vi "valve_control_output_tester.vi"(0 "STOP! Refnum":refnum<vi>, 2 "Voltage Arr Refnum":refnum<vi>, 3 "Startup Voltages":dbl[](array[numeric]), 4 "Liquid channel":tag="cDAQ1Mod4/ao3", 5 "Vapor channel":tag="cDAQ1Mod4/ao2") -> ()   [LabVIEW 2017]
uses:
  <vilib>/DAQmx/write.llb/DAQmx Write (Analog 1D Wfm NChan NSamp).vi
  <vilib>/DAQmx/create/channels.llb/DAQmx Create Channel (AO-Voltage-Basic).vi
  <vilib>/DAQmx/configure/timing.llb/DAQmx Timing (Sample Clock).vi
  <vilib>/DAQmx/miscellaneous.llb/DAQmx Fill In Error Info.vi
  <resource>/objmgr/daqmx.rc
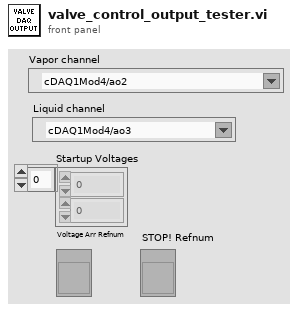
[diagram p1: front panel]
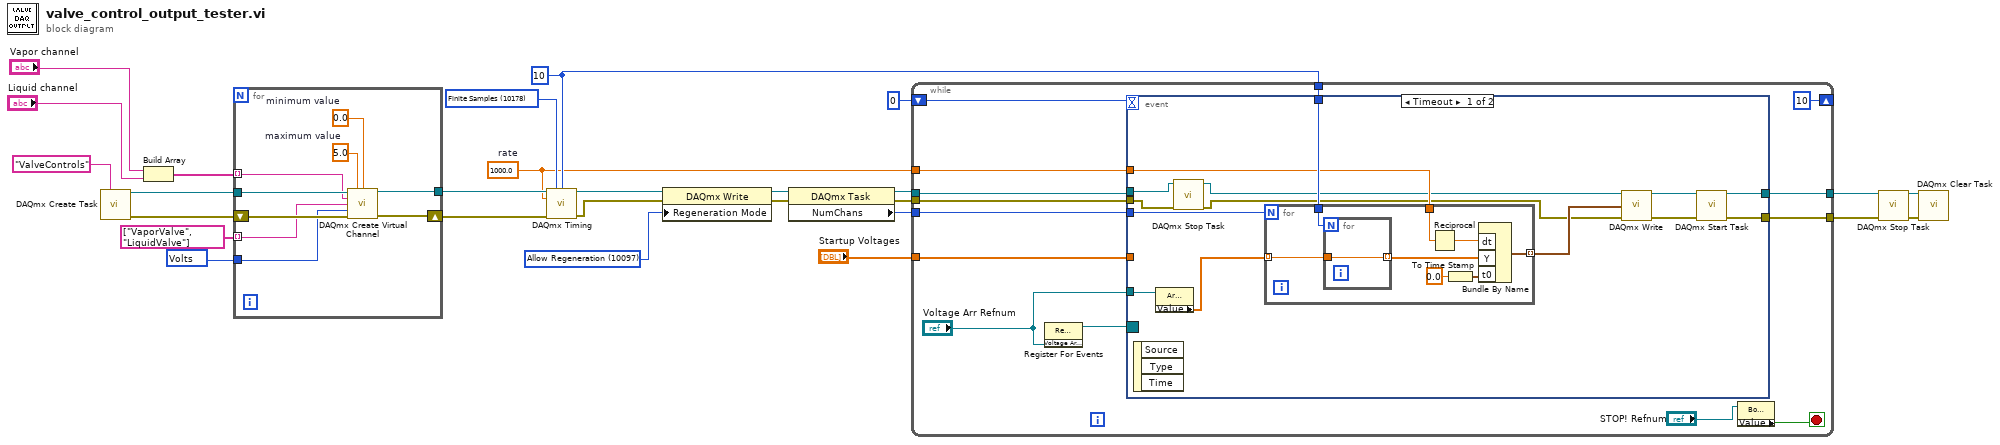
[diagram p0: block diagram]
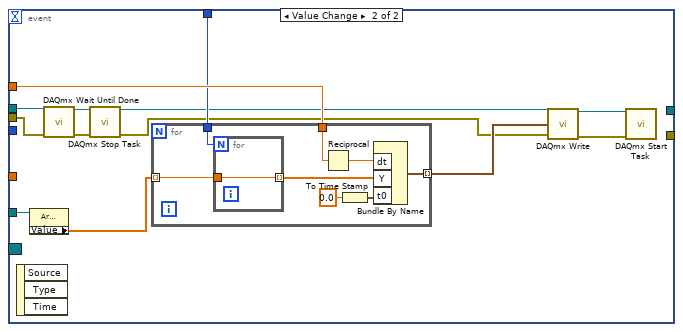
[diagram p2: hidden frame]
diagram:
  w14 = 10097 items=["Allow Regeneration"=10097, "Do Not Allow Regeneration"=10158] ("RegenMode")
  w9 = 10 ("samples per channel")
  w17 = 10178 items=["Finite Samples"=10178, "Continuous Samples"=10123, "Hardware Timed Single Point"=12522] ("sample mode")
  w8 = 1000.0  # rate
  w23 = 10348 items=["Volts"=10348, "From Custom Scale"=10065] ("units")
  n1 = call <vilib>:"DAQmx Create Task.vi"("new task name"="ValveControls") -> ("task out"=w26:refnum<k21>, "error out"=w25:errorcluster)  [unwired: 13 in]
  n2 = Build Array("Vapor channel", "Liquid channel") -> (w20:tag[])
  n3 = for {
    tunnel: w26 -> [w36]
    shift-right: [w28] -> w18
    shift-left: w25 -> [w35]
    tunnel: string[] ["VaporValve", "LiquidValve"] -> [w34] mode=indexing
    tunnel: w23 -> [w33]
    tunnel: w20 -> [w32] mode=indexing
    tunnel: [w29] -> w19
    w30 = 0.0  # minimum value
    w31 = 5.0  # maximum value
    n4 = call-poly <vilib>:"DAQmx Create Virtual Channel.vi"("task in"=w36, "maximum value"=w31, "minimum value"=w30, "physical channels"=w32, "name to assign"=w34, "units"=w33, "error in"=w35) -> ("task out"=w29:refnum<k21>, "error out"=w28:errorcluster)  [unwired: 7 in]
  }
  n5 = call-poly <vilib>:"DAQmx Timing.vi"("task/channels in"=w19, "sample mode"=w17, "samples per channel"=w9, "rate"=w8, "error in"=w18) -> ("task out"=w16:refnum<k21>, "error out"=w15:errorcluster)  [unwired: 9 in]
  n6 = property class="DAQmx Write"(reference=w16, error in=w15, "Regeneration Mode"=w14) -> (reference out=w13:refnum<k21>, error out=w12:errorcluster)
  n7 = property class="DAQmx Task"(reference=w13, error in=w12) -> (reference out=w7:refnum<k21>, error out=w6:errorcluster, "NumChans"=w11:u32)
  n8 = while {
    tunnel: w11 -> [w50]
    tunnel: "Startup Voltages" -> [w49]
    tunnel: w9 -> [w48]
    tunnel: w8 -> [w47]
    tunnel: w7 -> [w46]
    tunnel: [w44] -> w5
    tunnel: w6 -> [w45]
    tunnel: [w43] -> w4
    shift-right: [10] -> _
    shift-left: 0 -> [w41]
    stop <- w37 stop-if-true
    n9 = register-events("Voltage Arr Refnum") -> (reference out=w42:refnum<event-registration>)  [unwired: 2 in, 1 out]
    n10 = event shown="[0] Timeout" {
      selector: w42 -> [_ _]
      dyn-events: _ -> [_ _]
      timeout: w41 -> [_ _]
      tunnel: w50 -> [w64 _]
      tunnel: w49 -> [_ _]
      tunnel: w48 -> [w63 w82]
      tunnel: w47 -> [w62 w83]
      tunnel: w46 -> [w56 w81]
      tunnel: w45 -> [w55 w80]
      tunnel: [w58 _] -> w44
      tunnel: [w57 _] -> w43
      tunnel: "Voltage Arr Refnum" -> [w52 w79]
      event Timeout {
        n11 = event-data() -> ()  [unwired: 1 in, 3 out]
        n12 = property class="Arr (strict)"(reference=w52) -> ("Value"=w51:dbl[])  [unwired: 1 in, 2 out]
        n13 = call <vilib>:"DAQmx Stop Task.vi"("task/channels in"=w56, "error in"=w55) -> ("task out"=w54:refnum<k21>, "error out"=w53:errorcluster)  [unwired: 12 in]
        n14 = for {
          N: w64 -> [_]
          tunnel: [w72] -> w61 mode=indexing
          tunnel: w51 -> [w71] mode=indexing
          tunnel: w63 -> [w67]
          tunnel: w62 -> [w65]
          n15 = for {
            N: w67 -> [_]
            tunnel: w71 -> [w73]
            tunnel: [w73] -> w70 mode=indexing
          }
          n16 = Reciprocal(x=w65) -> (1/x=w66:dbl)
          n17 = To Time Stamp(1:0.0 ("number")) -> (0:w69:timestamp)
          n18 = Bundle By Name("dt"=w66, "Y"=w70, "t0"=w69) -> (w72:waveform(dbl))  [unwired: 1 out]
        }
        n19 = call-poly <vilib>:"DAQmx Write.vi"("task/channels in"=w54, "data"=w61, "error in"=w53) -> ("task out"=w60:refnum<k21>, "error out"=w59:errorcluster)  [unwired: 10 in, 1 out]
        n20 = call <vilib>:"DAQmx Start Task.vi"("task/channels in"=w60, "error in"=w59) -> ("task out"=w58:refnum<k21>, "error out"=w57:errorcluster)  [unwired: 12 in]
      }
      event Value Change {
        n21 = event-data() -> ()  [unwired: 1 in, 3 out]
        n22 = property class="Arr (strict)"(reference=w79) -> ("Value"=w78:dbl[])  [unwired: 1 in, 2 out]
        n23 = call <vilib>:"DAQmx Wait Until Done.vi"("task/channels in"=w81, "error in"=w80) -> ("task out"=w77:refnum<k21>, "error out"=w76:errorcluster)  [unwired: 12 in]
        n24 = call <vilib>:"DAQmx Stop Task.vi"("task/channels in"=w77, "error in"=w76) -> ("task out"=w74:refnum<k21>, "error out"=w75:errorcluster)  [unwired: 12 in]
        n25 = for {
          tunnel: [w94] -> w86 mode=indexing
          tunnel: w78 -> [w93] mode=indexing
          tunnel: w82 -> [w89]
          tunnel: w83 -> [w87]
          n26 = for {
            N: w89 -> [_]
            tunnel: w93 -> [w95]
            tunnel: [w95] -> w92 mode=indexing
          }
          n27 = Reciprocal(x=w87) -> (1/x=w88:dbl)
          n28 = To Time Stamp(1:0.0 ("number")) -> (0:w91:timestamp)
          n29 = Bundle By Name("dt"=w88, "Y"=w92, "t0"=w91) -> (w94:waveform(dbl))  [unwired: 1 out]
        }
        n30 = call-poly <vilib>:"DAQmx Write.vi"("task/channels in"=w74, "data"=w86, "error in"=w75) -> ("task out"=w85:refnum<k21>, "error out"=w84:errorcluster)  [unwired: 10 in, 1 out]
        n31 = call <vilib>:"DAQmx Start Task.vi"("task/channels in"=w85, "error in"=w84) -> ()  [unwired: 12 in, 2 out]
      }
    }
    n32 = property class="Bool (strict)"(reference="STOP! Refnum") -> ("Value"=w37:bool)  [unwired: 1 in, 2 out]
  }
  n33 = call <vilib>:"DAQmx Stop Task.vi"("task/channels in"=w5, "error in"=w4) -> ("task out"=w3:refnum<k21>, "error out"=w2:errorcluster)  [unwired: 12 in]
  n34 = call <vilib>:"DAQmx Clear Task.vi"("task in"=w3, "error in"=w2) -> ()  [unwired: 13 in, 1 out]
